vi "manifold config to odor count map (sub-vi).vi"(10 "manifold config array":T1) -> (2 "odor count map":T8)   [LabVIEW 2021]
uses:
  type-defs/odor channel to odor count map (type def).ctl
  type-defs/odor selection (type def).ctl
  type-defs/manifold configuration cluster array (type def).ctl
  type-defs/manifold configuration cluster (type def).ctl
  type-defs/manifold selection.ctl
  type-defs/single port single odor cluster.ctl
  type-defs/port number (type def).ctl
  type-defs/odor color (type def).ctl
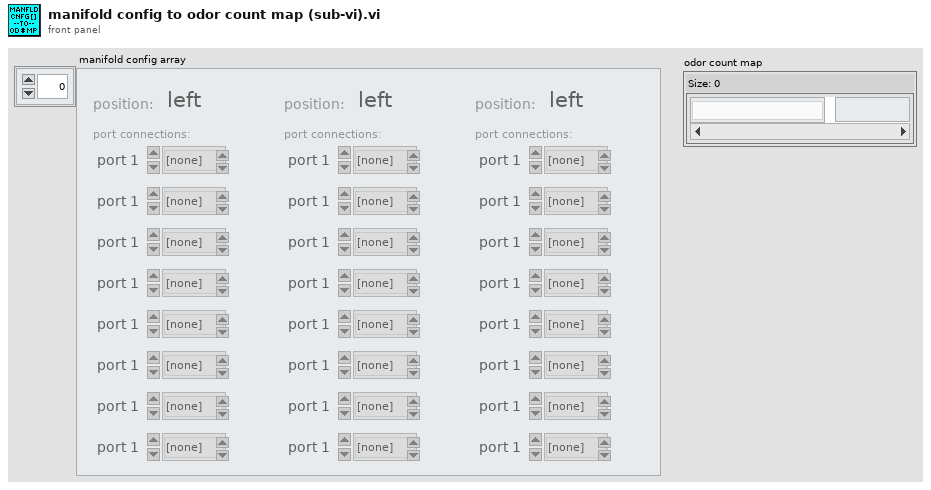
[diagram p1: front panel]
types:
  T1 = typedef "manifold configuration cluster array (type def).ctl" = T2[]
  T2 = typedef "manifold configuration cluster (type def).ctl" = cluster{"position:":T3, "port connections:":T4[]}
  T3 = typedef "manifold selection.ctl" = enum16{"left", "middle", "right"}
  T4 = typedef "single port single odor cluster.ctl" = cluster{"port number":T5, "connected odor":T6, "error":bool, "odor color":T7}
  T5 = typedef "port number (type def).ctl" = enum16{"port 1", "port 2", "port 3", "port 4", "port 5", "port 6", "port 7", "port 8"}
  T6 = typedef "odor selection (type def).ctl" = enum16{"[none]", "odor 1", "odor 2", "odor 3", "odor 4", "odor 5", "odor 6", "odor 7", "odor 8", "odor 9", "odor 10"}
  T7 = typedef "odor color (type def).ctl" = u16
  T8 = typedef "odor channel to odor count map (type def).ctl" = map{T6, u16}
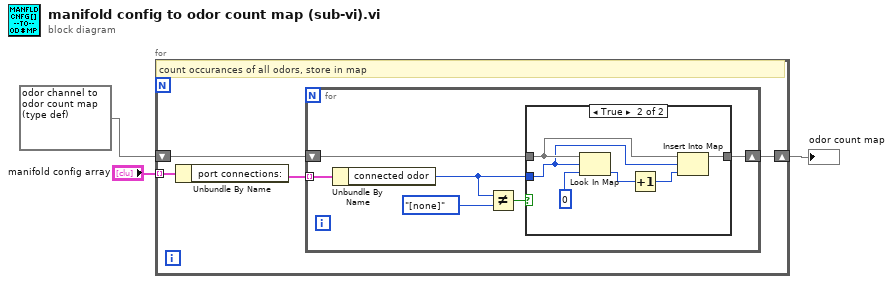
[diagram p0: block diagram]
diagram:
  n1 = for {
    tunnel: "manifold config array" -> [w6] mode=indexing
    shift-right: [w4] -> w2
    shift-left: T8 {} -> [w5]
    # "count occurances of all odors, store in map"
    n2 = Unbundle By Name(w6) -> ("port connections:"=w7:T4[])
    n3 = for {
      tunnel: w7 -> [w13] mode=indexing
      shift-right: [w12] -> w4
      shift-left: w5 -> [w11]
      n4 = Unbundle By Name(w13) -> ("connected odor"=w10:T6)
      n5 = Not Equal?(x=w10, y=odor_selection_(type_def)."[none]" ("connected odor")) -> (x != y?=w8:bool)
      n6 = case shown="True" w8 {
        tunnel: [w14 w16] -> w12
        tunnel: w11 -> [w14 w17]
        tunnel: w10 -> [_ w15]
        frame False {
        }
        frame True {
          n7 = Look In Map(map=w17, key=w15, default value=u16 0) -> (value=w18:u16)  [unwired: 1 out]
          n8 = Increment(x=w18) -> (x+1=w19:u16)
          n9 = Insert Into Map(map in=w17, key=w15, value=w19) -> (map out=w16:T8)  [unwired: 2 out]
        }
      }
    }
  }
  "odor count map" <- w2
